vi "DB_查询通讯表.vi"(8 "error in (no error)":errorcluster caption="错误输入（无错误）", 10 "ID":i32) -> (0 "error out":errorcluster caption="错误输出", 2 "设备通讯参数":T1={"设备站号"=1, "IP Addr"="127.0.0.1", "Port"=255, "COM"="COM3", "baud rate (9600)"=9600, "Protocol"=enum."Serial Port"})   [LabVIEW 2018]
uses:
  <vilib>/drjdpowell/SQLite Library/SQL Connection/Connection.lvclass
  <vilib>/drjdpowell/SQLite Library/SQL Statement/SQL Statement.lvclass/SQL Statement.ctl
  <vilib>/drjdpowell/SQLite Library/SQL Connection/Open (path).vi
  <vilib>/drjdpowell/SQLite Library/SQL Statement/Bind Integer.vi
  <vilib>/drjdpowell/SQLite Library/SQL Statement/Column I64.vi
  <vilib>/JDP Science/JDP Science Common Utilities/Trim Whitespace__JDP.vi
  <vilib>/drjdpowell/SQLite Library/SQL Connection/Open (string).vi
  <vilib>/AdvancedString/Path To Command Line String.vi
  <vilib>/drjdpowell/SQLite Library/SQL Statement/Error Message.vi
  <vilib>/drjdpowell/SQLite Library/SQL Statement/Column String.vi
  <vilib>/drjdpowell/SQLite Library/SQLite.lvlib
  <vilib>/drjdpowell/SQLite Library/SQL Statement/SQL Statement.lvclass
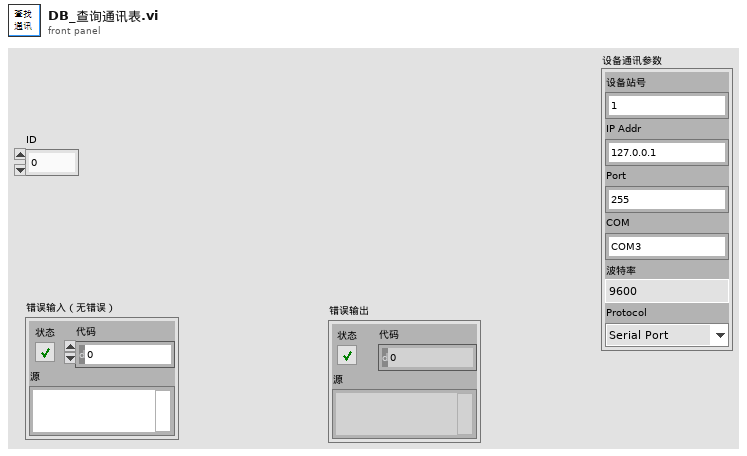
[diagram p1: front panel]
types:
  T1 = cluster{"设备站号":u8, "IP Addr":string, "Port":u16, "COM":string, "baud rate (9600)":u32, "Protocol":enum16{"Serial Port", "Modbus TCP/IP"}}
  T2 = enum16{"New or existing", "Existing", "Read only"}
  T3 = cluster{"设备站号":u8, "IP Addr":string, "Port":u16, "COM":string, "baud rate (9600)":u32, "控制方式":enum16{"Serial Port", "Modbus TCP/IP"}}
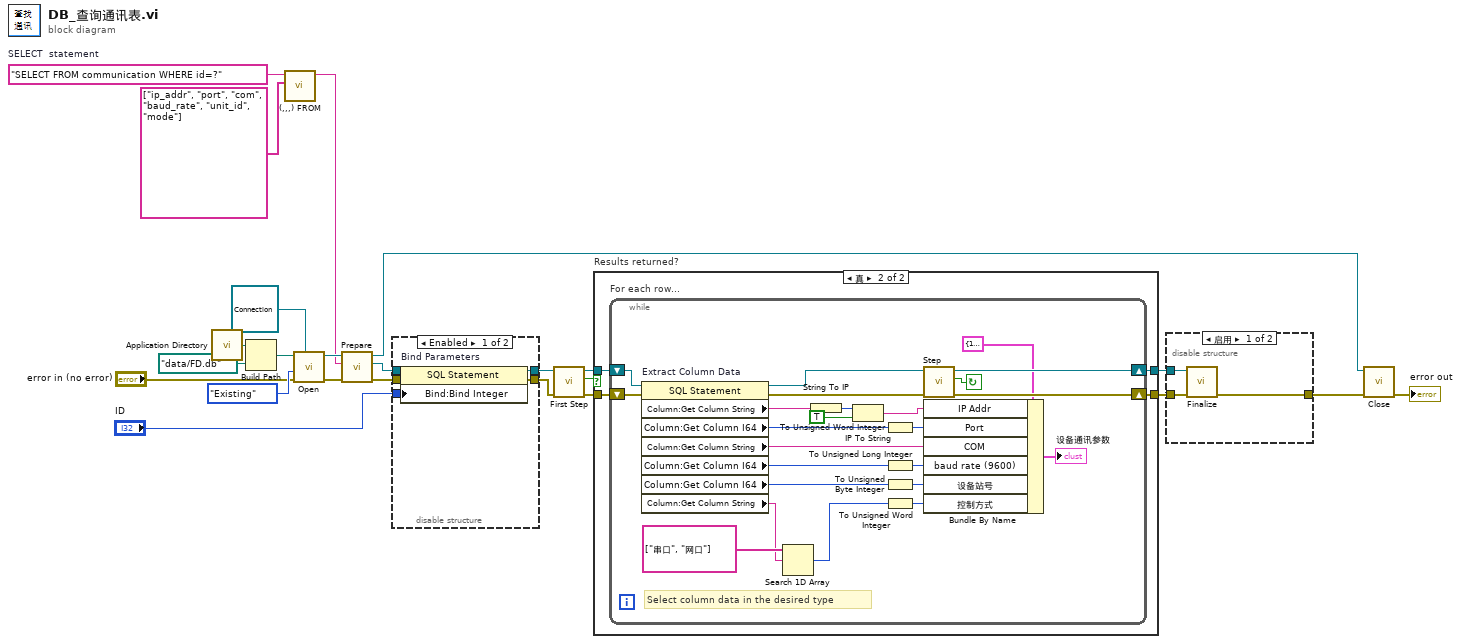
[diagram p0: block diagram]
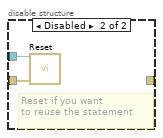
[diagram p2: hidden frame]
diagram:
  w17 = "SELECT FROM communication WHERE id=?"  # SELECT  statement
  n1 = call <vilib>:"Application Directory.vi"() -> ("Application Directory"=w24:path)
  n2 = Build Path(base path=w24, name or relative path=path "data/FD.db" ("Application Directory")) -> (appended path=w22:path)
  n3 = call <vilib>:"(,,,) FROM.vi"("Column Names"=string[] ["ip_addr", "port", "com", "baud_rate", "unit_id", "mode"] ("列首字符串[]"), "SQL containing FROM clause"=w17) -> ("SQL"=w1:string)  [unwired: 9 in]
  n4 = call-poly <vilib>:"Open.vi"("SQLite Connection type"=refnum<class "Connection.lvclass"> refnum, "error in (no error)"="error in (no error)", "File Option"=T2."Existing", "db file"=w22) -> ("error out"=w5:errorcluster, "SQLite Connection"=w4:refnum<class "Connection.lvclass">)  [unwired: 6 in]
  n5 = call <vilib>:"Prepare.vi"("error in (no error)"=w5, "SQL"=w1, "SQLite Connection in"=w4) -> ("error out"=w13:errorcluster, "SQL Statement"=w10:refnum<class "SQL Statement.lvclass">, "SQLite Connection"=w2:refnum<class "Connection.lvclass">)  [unwired: 4 in, 2 out]
  n6 = disable-structure shown="Enabled" {
    disable-tunnel: w10 -> [w29 w31]
    disable-tunnel: [w28 w31] -> w11
    disable-tunnel: [w27 w30] -> w12
    disable-tunnel: w13 -> [w26 w30]
    disable-tunnel: "ID" -> [w25 _]
    frame Enabled {
      n7 = property on="Bind Parameters" class="SQL Statement"(reference=w29, error in=w26, "Bind:Bind Integer"=w25) -> (reference out=w28:refnum<class "SQL Statement.lvclass">, error out=w27:errorcluster)
    }
    frame Disabled {
    }
  }
  n8 = call <vilib>:"First Step.vi"("error in (no error)"=w12, "SQL Statement in"=w11) -> ("error out"=w8:errorcluster, "Row returned"=w7:bool, "SQL Statement"=w9:refnum<class "SQL Statement.lvclass">)  [unwired: 7 in]
  n9 = case "Results returned?" shown="真" w7 {
    tunnel: [w33 w37] -> w14
    tunnel: [w32 w36] -> w15
    tunnel: w9 -> [w33 w35]
    tunnel: w8 -> [w32 w34]
    frame False {
    }
    frame True {
      n10 = while "For each row..." {
        shift-right: [w60] -> w37
        shift-left: w35 -> [w57]
        shift-right: [w58] -> w36
        shift-left: w34 -> [w56]
        stop <- w55 continue-if-true
        # "Select column data in the desired type"
        n11 = property on="Extract Column Data" class="SQL Statement"(reference=w57, error in=w56) -> (reference out=w61:refnum<class "SQL Statement.lvclass">, error out=w59:errorcluster, "Column:Get Column String"=w43:string, "Column:Get Column I64"=w54:i64, "Column:Get Column String"=w47:string, "Column:Get Column I64"=w48:i64, "Column:Get Column I64"=w44:i64, "Column:Get Column String"=w51:string)
        n12 = Search 1D Array(1D array=string[] ["串口", "网口"], element=w51) -> (index of element=w50:i32)  [unwired: 1 in]
        n13 = String To IP(1:w43) -> (0:w41:u32)
        n14 = IP To String(1:TRUE ("句点符号？(F)"), 2:w41) -> (0:w40:string)
        n15 = To Unsigned Word Integer(number=w54) -> (unsigned 16bit integer=w53:u16)
        n16 = To Unsigned Long Integer(number=w48) -> (unsigned 32bit integer=w49:u32)
        n17 = To Unsigned Byte Integer(number=w44) -> (unsigned 8bit integer=w45:u8)
        n18 = To Unsigned Word Integer(number=w50) -> (unsigned 16bit integer=w46:u16)
        n19 = call <vilib>:"Step.vi"("error in (no error)"=w59, "SQL Statement in"=w61) -> ("error out"=w58:errorcluster, "Row returned"=w55:bool, "SQL Statement"=w60:refnum<class "SQL Statement.lvclass">)  [unwired: 7 in]
        n20 = Bundle By Name(cluster=T3 {"设备站号"=1, "IP Addr"="127.0.0.1", "Port"=255, "COM"="COM3", "baud rate (9600)"=9600, "控制方式"=enum."Serial Port"} ("设备通讯参数"), "IP Addr"=w40, "Port"=w53, "COM"=w47, "baud rate (9600)"=w49, "设备站号"=w45, "控制方式"=w46) -> (→"设备通讯参数":T3)
      }
    }
  }
  n21 = disable-structure shown="启用" {
    disable-tunnel: w14 -> [w64 w66]
    disable-tunnel: w15 -> [w63 w65]
    disable-tunnel: [w62 _] -> w3
    frame Enabled {
      n22 = call <vilib>:"Finalize.vi"("error in (no error)"=w63, "SQL Statement in"=w64) -> ("error out"=w62:errorcluster)  [unwired: 9 in]
    }
    frame Disabled {
      # "Reset if you want\nto reuse the statement"
      n23 = call <vilib>:"Reset.vi"("error in (no error)"=w65, "SQL Statement in"=w66) -> ()  [unwired: 8 in, 2 out]
    }
  }
  n24 = call-dynamic "Close.vi"("error in (no error)"=w3, "SQLite Connection in"=w2) -> ("error out"=→"error out":errorcluster)  [unwired: 9 in]
